vi "Conditions.vi"(11 "Transition Config in":refnum<class "Transition Config.lvclass">) -> (1 "Conditions":refnum<class "Condition Config.lvclass">[](array[class]), 2 "Logic":T1)   [LabVIEW 2020, in "VolatusSeqConfig.lvlib" / "Transition Config.lvclass"]
uses:
  Transition Config.lvclass
  Transition Config.lvclass/Transition Config.ctl
  Condition Config/Condition Config.lvclass
  Condition Logic.ctl
  VolatusSeqConfig.lvlib
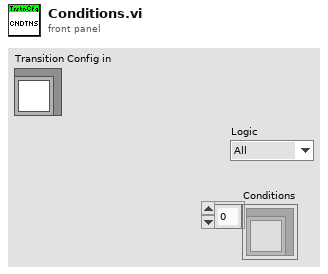
[diagram p1: front panel]
types:
  T1 = typedef "VolatusSeqConfig.lvlib/Condition Logic.ctl" = enum16{"All", "Any"}
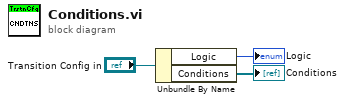
[diagram p0: block diagram]
diagram:
  n1 = Unbundle By Name("Transition Config in") -> ("Logic"=→"Logic":T1, "Conditions"=→"Conditions":refnum<class "Condition Config.lvclass">[])
